vi "Get Last Error Terminal on Error-Chained Create User Events.vi"(8 "error in (no error)":errorcluster, 11 "VI in":refnum<vi>) -> (0 "error out":errorcluster, 1 "Connected Sink Terminals":refnum<vi>[](array[refnum]), 2 "Last Error Source Terminal":refnum<vi>, 3 "VI out":refnum<vi>)   [LabVIEW 2018, in "Scripting.lvlib"]
uses:
  Scripting.lvlib
  <vilib>/Utility/traverseref.llb/TRef TravTarget.ctl
  <vilib>/Utility/traverseref.llb/VI Scripting - Traverse.lvlib
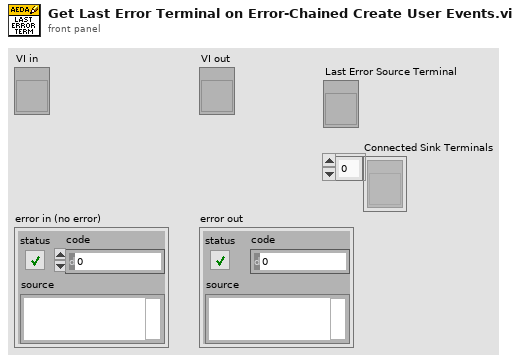
[diagram p1: front panel]
types:
  T1 = typedef "TRef TravTarget.ctl" = enum16{"FP", "BD", "Other"}
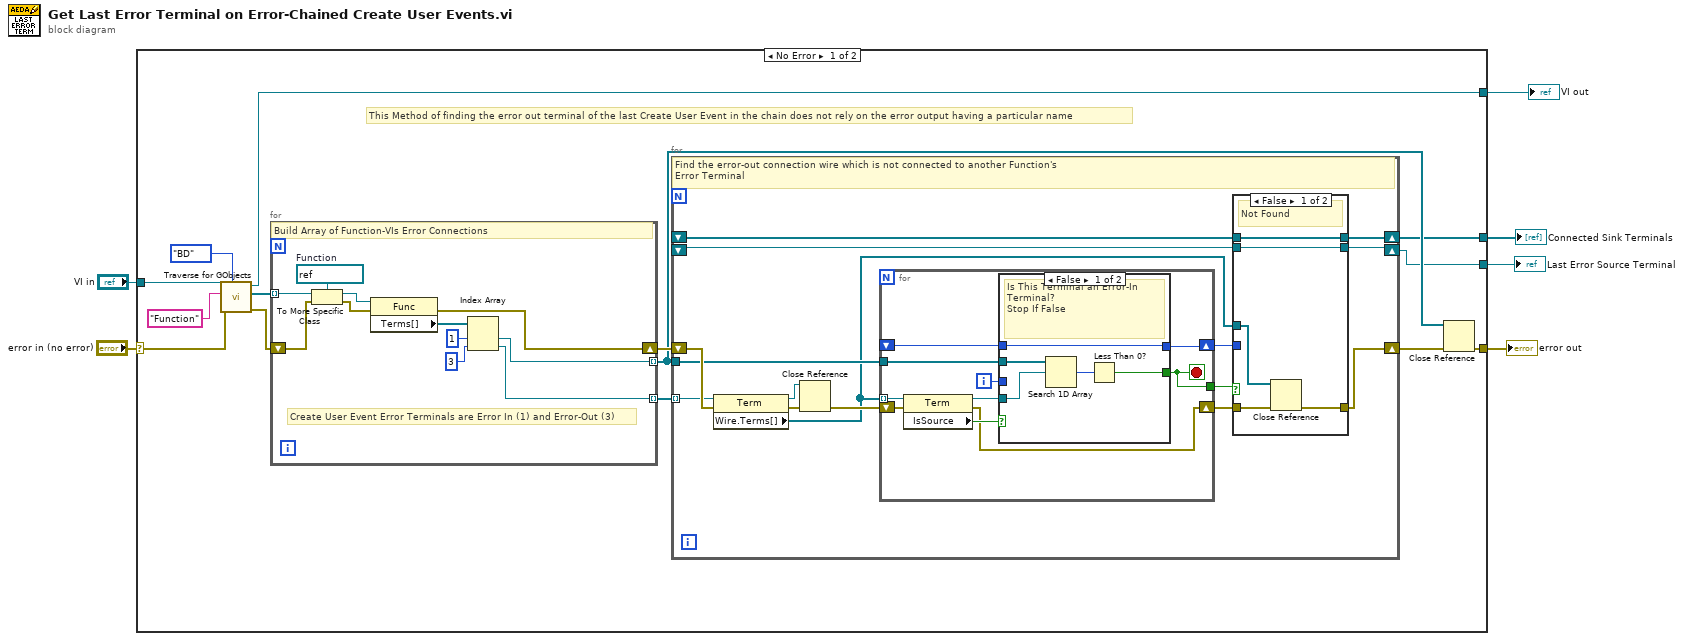
[diagram p0: block diagram]
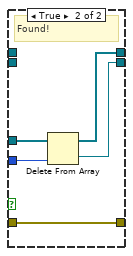
[diagram p3: hidden frame]
diagram:
  n1 = case shown="No Error" "error in (no error)" {
    selector: "error in (no error)" -> [w13 w74]
    tunnel: "VI in" -> [w14 w73]
    tunnel: [w10 _] -> w4
    tunnel: [w9 _] -> w3
    tunnel: [w8 w74] -> w2
    tunnel: [w7 w73] -> w1
    frame No Error {
      # "This Method of finding the error out terminal of the last Create User Event in the chain does not rely on the error output having a particular name"
      n2 = call <vilib>:"Traverse for GObjects.vi"("Traverse Target"=TRef_TravTarget."BD", "error in (no error)"=w13, "Class Name"="Function", "VI Refnum"=w14) -> ("error out"=w18:errorcluster, "References"=w17:refnum<vi>[], "dup VI Refnum"=w7:refnum<vi>)  [unwired: 4 in, 1 out]
      n3 = for {
        tunnel: w17 -> [w31] mode=indexing
        tunnel: [w21] -> w11 mode=indexing
        tunnel: [w23] -> w19 mode=indexing
        shift-right: [w22] -> w20
        shift-left: w18 -> [w29]
        w27 = refnum<vi> refnum  # Function
        # "Create User Event Error Terminals are Error In (1) and Error-Out (3)"
        # "Build Array of Function-VIs Error Connections"
        n4 = To More Specific Class(target class=w27, reference=w31, error in=w29) -> (specific class reference=w30:refnum<vi>, error out=w28:errorcluster)
        n5 = property class="Func"(reference=w30, error in=w28) -> (error out=w22:errorcluster, "Terms[]"=w26:refnum<vi>[])  [unwired: 1 out]
        n6 = Index Array(array=w26, index #1=1 ("index"), index #2=3 ("index")) -> (element #1=w21:refnum<vi>, element #2=w23:refnum<vi>)
      }
      n7 = for {
        tunnel: w19 -> [w45] mode=indexing
        shift-right: [w32] -> w12
        shift-left: w20 -> [w46]
        tunnel: w11 -> [w41]
        shift-right: [w37] -> w9
        shift-left: _ -> [w34]
        shift-right: [w36] -> w10
        shift-left: _ -> [w35]
        # "Find the error-out connection wire which is not connected to another Function's\nError Terminal"
        n8 = property class="Term"(reference=w45, error in=w46) -> (reference out=w43:refnum<vi>, error out=w44:errorcluster, "Wire.Terms[]"=w39:refnum<vi>[])
        n9 = Close Reference(reference=w43, error in (no error)=w44) -> (error out=w42:errorcluster)
        n10 = for {
          tunnel: w39 -> [w56] mode=indexing
          shift-right: [w50] -> w33
          shift-left: w42 -> [w55]
          tunnel: w41 -> [w53]
          tunnel: [w51] -> w40
          shift-right: [w48] -> w38
          shift-left: _ -> [w47]
          i -> [w49]
          stop <- w51 stop-if-true
          n11 = property class="Term"(reference=w56, error in=w55) -> (reference out=w52:refnum<vi>, error out=w50:errorcluster, "IsSource"=w54:bool)
          n12 = case shown="False" w54 {
            tunnel: w53 -> [w61 _]
            tunnel: w52 -> [w60 _]
            tunnel: [w58 _] -> w51
            tunnel: w49 -> [_ w62]
            tunnel: [w57 w62] -> w48
            tunnel: w47 -> [w57 _]
            frame False {
              # "Is This Terminal an Error-In Terminal?\nStop If False"
              n13 = Search 1D Array(1D array=w61, element=w60) -> (index of element=w59:i32)  [unwired: 1 in]
              n14 = Less Than 0?(x=w59) -> (x < 0?=w58:bool)
            }
            frame True {
              # "Store Source Terminal"
              # "Source \nCannot be an Error-In Terminal"
            }
          }
        }
        n15 = case shown="False" w40 {
          tunnel: w39 -> [w65 w72]
          tunnel: w38 -> [_ w71]
          tunnel: [w66 w70] -> w37
          tunnel: [w67 w69] -> w36
          tunnel: w35 -> [w67 _]
          tunnel: w34 -> [w66 _]
          tunnel: w33 -> [w64 w68]
          tunnel: [w63 w68] -> w32
          frame False {
            # "Not Found"
            n16 = Close Reference(reference=w65, error in (no error)=w64) -> (error out=w63:errorcluster)
          }
          frame True {
            # "Found!"
            n17 = Delete From Array(array=w72, index=w71) -> (deleted portion=w69:refnum<vi>, array with subset deleted=w70:refnum<vi>[])  [unwired: 1 in]
          }
        }
      }
      n18 = Close Reference(reference=w11, error in (no error)=w12) -> (error out=w8:errorcluster)
    }
    frame Error {
    }
  }
  "error out" <- w2
  "Last Error Source Terminal" <- w4
  "Connected Sink Terminals" <- w3
  "VI out" <- w1
